vi "constant speed using encoder.vi"(2 "s78_2":i16, 3 "s78_1":i16, 4 "s77_2":i16, 5 "s77_1":i16) -> ()   [LabVIEW 2018]
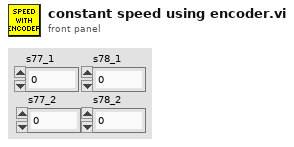
[diagram p1: front panel]
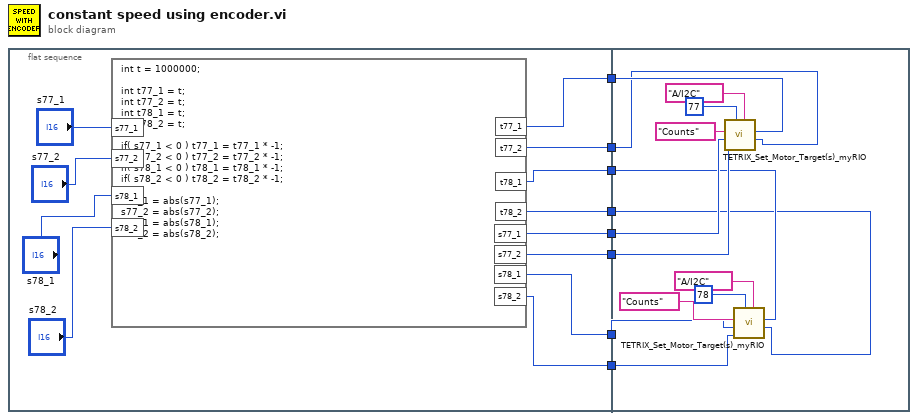
[diagram p0: block diagram]
diagram:
  n1 = flat-sequence {
    tunnel: [w16] -> w8
    tunnel: [w15] -> w7
    tunnel: [w14] -> w6
    tunnel: [w13] -> w5
    tunnel: [w12] -> w4
    tunnel: [w11] -> w3
    tunnel: [w10] -> w2
    tunnel: [w9] -> w1
    tunnel: w8 -> [w28]
    tunnel: w7 -> [w27]
    tunnel: w6 -> [w26]
    tunnel: w5 -> [w25]
    tunnel: w4 -> [w24]
    tunnel: w3 -> [w23]
    tunnel: w2 -> [w22]
    tunnel: w1 -> [w21]
    frame #0 {
      n2 = formula code="int t = 1000000;\n\nint t77_1 = t;\nint t77_2 = t;\nint t78_1 = t;\nint t78_2 = t;\n\nif( s77_1 < 0 ) t77_1 = t77_1 * -1;\nif( s77_2 < 0 ) t77_2 = t77_2 * -1;\nif( s78_1 < 0 ) t78_1 = t78_1 * -1;\nif( s78_2 < 0 ) t78_2 = t78_2 * -1;\n\ns77_1 = abs(s77_1);\ns77_2 = abs(s77_2);\ns78_1 = abs(s78_1);\ns78_2 = abs(s78_2);"("s77_1"="s77_1", "s77_2"="s77_2", "s78_1"="s78_1", "s78_2"="s78_2") -> ("t77_1"=w12:i32, "t77_2"=w11:i32, "t78_1"=w10:i32, "t78_2"=w9:i32, "s77_1"=w16:i16, "s77_2"=w15:i16, "s78_1"=w14:i16, "s78_2"=w13:i16)
    }
    frame #1 {
      n3 = call <vilib>:"TETRIX_Set_Motor_Target(s)_myRIO.vi"("Motor 2 Encoder Target"=w23, "Motor 1 Encoder Target"=w24, "myRIO MXP Port A/B"=tag "A/I2C", "Controller ID#  (I2C Address)"=u8 77, "Motor 2 Constant Speed (Degrees per Second)"=w27, "Motor 1 Contant Speed (Degrees per Second)"=w28, "Encoder Units"="Counts") -> ()  [unwired: 2 in, 1 out]
      n4 = call <vilib>:"TETRIX_Set_Motor_Target(s)_myRIO.vi"("Motor 2 Encoder Target"=w21, "Motor 1 Encoder Target"=w22, "myRIO MXP Port A/B"=tag "A/I2C", "Controller ID#  (I2C Address)"=u8 78, "Motor 2 Constant Speed (Degrees per Second)"=w25, "Motor 1 Contant Speed (Degrees per Second)"=w26, "Encoder Units"="Counts") -> ()  [unwired: 2 in, 1 out]
    }
  }
